vi "Search For NodePathArray Item by Index.vi"(1 "index of NodePathArray":i32, 2 "NodePathArray":string[](array[string]), 3 "Items to search":string[](array[string])) -> (0 "result":i32)   [LabVIEW 2011]
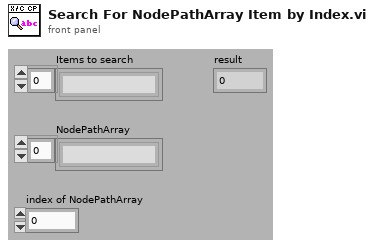
[diagram p1: front panel]
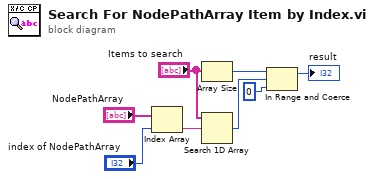
[diagram p0: block diagram]
diagram:
  n1 = Index Array(array="NodePathArray", index="index of NodePathArray") -> (element=w2:string)
  n2 = Array Size(array="Items to search") -> (size(s)=w5:i32)
  n3 = Search 1D Array(1D array="Items to search", element=w2) -> (index of element=w3:i32)  [unwired: 1 in]
  n4 = In Range and Coerce(upper limit=w5, x=w3, lower limit=0) -> (coerced(x)=→"result":i32)  [unwired: 1 out]
